vi "Data Socket panel  Reader-2.vi"() -> ()   [LabVIEW 2012]
doc: "© Copyright M. Ferrari 2012 \n[LV 2009]"
panel:
  in  "stop":bool
  out "Waveform Chart":dbl(graph)
  # "DATA SOCKET SUBSCRIBER (READER)"
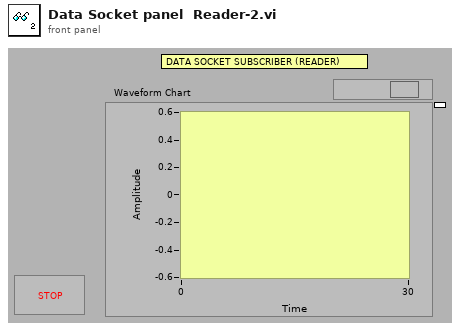
[diagram p1: front panel]
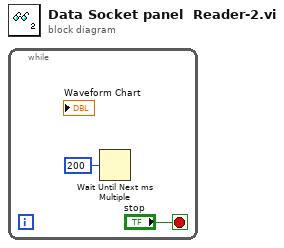
[diagram p0: block diagram]
diagram:
  n1 = while {
    stop <- "stop" stop-if-true
    n2 = Wait Until Next ms Multiple(millisecond multiple=u32 200) -> ()  [unwired: 1 out]
  }
